vi "XY Graph Multiple TipStrip Event Registration.vi"(8 "Error In":errorcluster, 11 "XY Graph Refnums":refnum<vi>[](array[refnum])) -> (0 "Error Out":errorcluster, 3 "Tipstrips Event Registrations":refnum<event-registration>[](array[refnum]))   [LabVIEW 2021, in "XY Graph Add-Ons.lvlib"]
uses:
  XY Graph/XY Graph Add-Ons.lvlib
  XY Graph/XY Graph Refnum.ctl
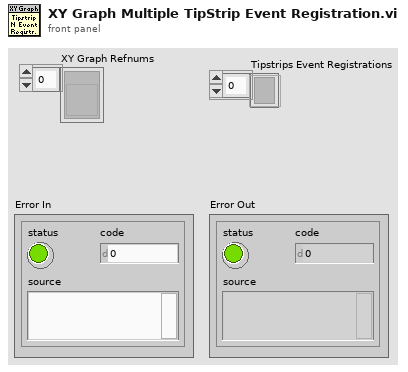
[diagram p1: front panel]
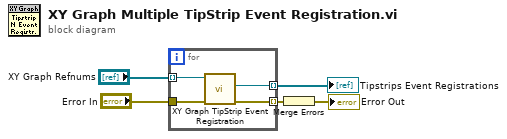
[diagram p0: block diagram]
diagram:
  n1 = for {
    tunnel: "XY Graph Refnums" -> [w9] mode=indexing
    tunnel: "Error In" -> [w8]
    tunnel: [w7] -> w1 mode=indexing
    tunnel: [w6] -> w3 mode=indexing
    n2 = call "XY Graph TipStrip Event Registration.vi"("error in (no error)"=w8, "XY Graph Refnum"=w9) -> ("error out"=w6:errorcluster, "Event Registration Refnum"=w7:refnum<event-registration>)  [unwired: 7 in, 1 out]
  }
  "Tipstrips Event Registrations" <- w1
  n3 = Merge Errors(w3) -> (→"Error Out":errorcluster)
